vi "Save VI.vi"(8 "error in (no error)":errorcluster, 10 "Ctl Properties":T1[](array[typedef]), 11 "VI Properties":T2) -> (0 "error out":errorcluster, 2 "Saved?":bool, 3 "VI out":refnum<vi>)   [LabVIEW 2023, in "VI Properties Editor.lvlib"]
doc: "Saves a VI based with <B>VI Properties</B> and <B>Ctl Properties</B>."
uses:
  CTLs/VI Properties.ctl
  <vilib>/picture/picture.llb/imagedata.ctl
  CTLs/Control Properties.ctl
  VI Properties Editor.lvlib
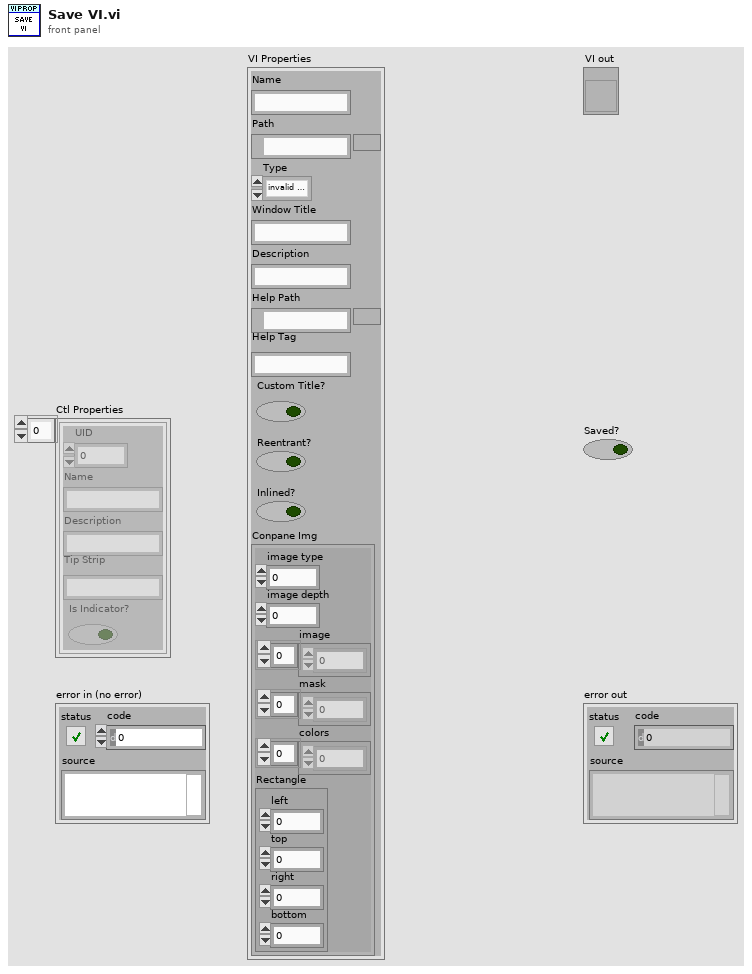
[diagram p1: front panel]
types:
  T1 = typedef "VI Properties Editor.lvlib/Control Properties.ctl" = cluster{"UID":i32, "Name":string, "Description":string, "Tip Strip":string, "Is Indicator?":bool}
  T2 = typedef "VI Properties Editor.lvlib/VI Properties.ctl" = cluster{"Name":string, "Path":path, "Type":enum32{"invalid VI type", "Standard VI", "Control VI", "Global VI", "Polymorphic VI", "Configuration VI", "SubSystem", "Facade VI", "Method VI", "Statechart Diagram VI"}, "Window Title":string, "Description":string, "Help Path":path, "Help Tag":string, "Custom Title?":bool, "Reentrant?":bool, "Inlined?":bool, "Conpane Img":T3}
  T3 = typedef "imagedata.ctl" = cluster{"image type":i32, "image depth":i32, "image":u8[], "mask":u8[], "colors":u32[], "Rectangle":cluster{"left":i16, "top":i16, "right":i16, "bottom":i16}}
  T4 = enum32{"invalid VI type", "Standard VI", "Control VI", "Global VI", "Polymorphic VI", "Configuration VI", "SubSystem", "Facade VI", "Method VI", "Statechart Diagram VI"}
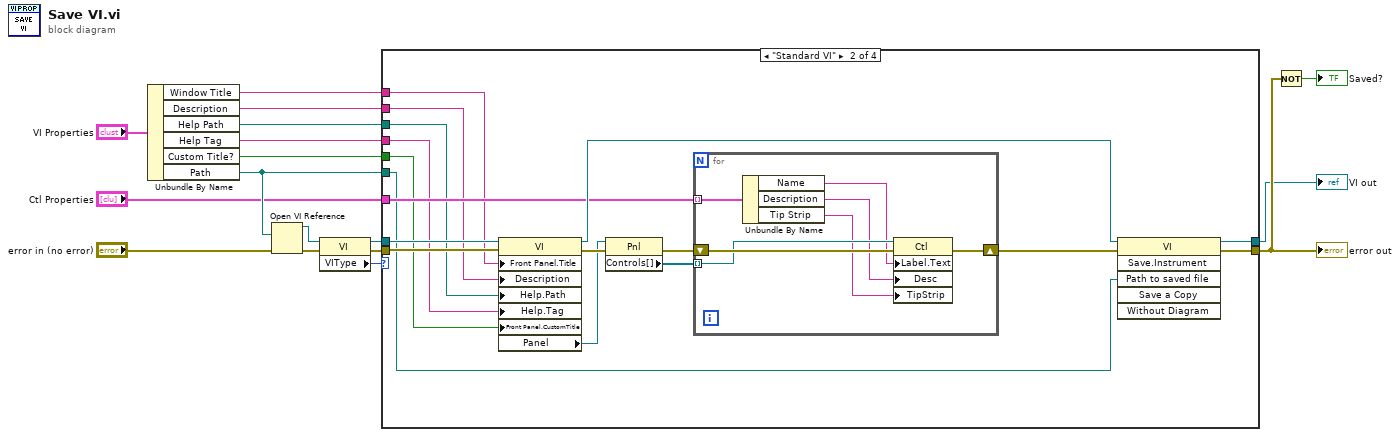
[diagram p0: block diagram]
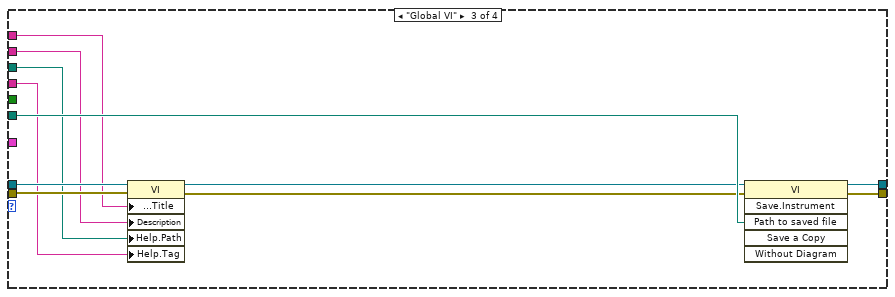
[diagram p3: hidden frame]
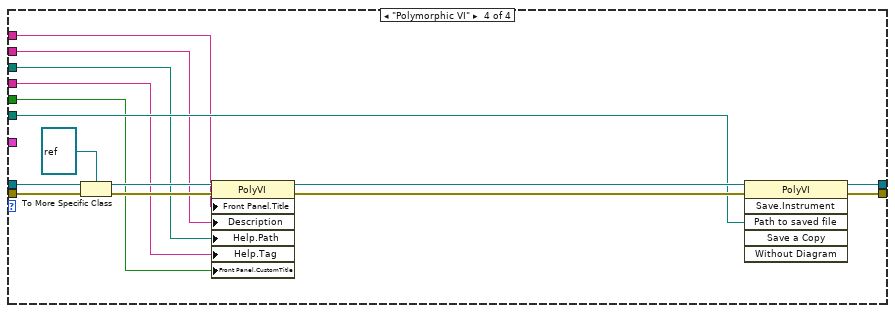
[diagram p4: hidden frame]
diagram:
  n1 = Unbundle By Name("VI Properties") -> ("Window Title"=w2:string, "Description"=w5:string, "Help Path"=w4:path, "Help Tag"=w6:string, "Custom Title?"=w1:bool, "Path"=w7:path)
  n2 = Open VI Reference(vi path=w7, error in (no error)="error in (no error)") -> (vi reference=w10:refnum<vi>, error out=w13:errorcluster)  [unwired: 4 in]
  n3 = property class="VI"(reference=w10, error in=w13) -> (reference out=w11:refnum<vi>, error out=w12:errorcluster, "VIType"=w14:T4)
  n4 = case shown="\"Standard VI\"" w14 {
    tunnel: [w18 w36 w54 w69] -> w15
    tunnel: [w19 w35 w53 w68] -> w16
    tunnel: w11 -> [w18 w28 w49 w66]
    tunnel: w12 -> [w19 w27 w48 w65]
    tunnel: w5 -> [_ w25 w45 w56]
    tunnel: w6 -> [_ w23 w47 w57]
    tunnel: w4 -> [_ w22 w46 w58]
    tunnel: w7 -> [_ w21 w52 w60]
    tunnel: "Ctl Properties" -> [_ w26 _ _]
    tunnel: w2 -> [_ w24 w44 w55]
    tunnel: w1 -> [_ w20 _ w59]
    frame "invalid VI type", Default {
    }
    frame "Standard VI" {
      n5 = property class="VI"(reference=w28, error in=w27, "Front Panel.Title"=w24, "Description"=w25, "Help.Path"=w22, "Help.Tag"=w23, "Front Panel.CustomTitle"=w20) -> (reference out=w31:refnum<vi>, error out=w34:errorcluster, "Panel"=w33:refnum<vi>)
      n6 = property class="Pnl"(reference=w33, error in=w34) -> (error out=w29:errorcluster, "Controls[]"=w30:refnum<vi>[])  [unwired: 1 out]
      n7 = for {
        tunnel: w30 -> [w41] mode=indexing
        shift-right: [w43] -> w32
        shift-left: w29 -> [w42]
        tunnel: w26 -> [w40] mode=indexing
        n8 = Unbundle By Name(w40) -> ("Name"=w39:string, "Description"=w38:string, "Tip Strip"=w37:string)
        n9 = property class="Ctl"(reference=w41, error in=w42, "Label.Text"=w39, "Desc"=w38, "TipStrip"=w37) -> (error out=w43:errorcluster)  [unwired: 1 out]
      }
      n10 = invoke class="VI" method="Save.Instrument"(reference=w31, error in=w32, "Path to saved file"=w21) -> (reference out=w36:refnum<vi>, error out=w35:errorcluster)  [unwired: 3 in, 4 out]
    }
    frame "Global VI" {
      n11 = property class="VI"(reference=w49, error in=w48, "Front Panel.Title"=w44, "Description"=w45, "Help.Path"=w46, "Help.Tag"=w47) -> (reference out=w50:refnum<vi>, error out=w51:errorcluster)
      n12 = invoke class="VI" method="Save.Instrument"(reference=w50, error in=w51, "Path to saved file"=w52) -> (reference out=w54:refnum<vi>, error out=w53:errorcluster)  [unwired: 3 in, 4 out]
    }
    frame "Polymorphic VI" {
      n13 = To More Specific Class(target class=refnum<vi> refnum, reference=w66, error in=w65) -> (specific class reference=w64:refnum<vi>, error out=w63:errorcluster)
      n14 = property class="PolyVI"(reference=w64, error in=w63, "Front Panel.Title"=w55, "Description"=w56, "Help.Path"=w58, "Help.Tag"=w57, "Front Panel.CustomTitle"=w59) -> (reference out=w62:refnum<vi>, error out=w61:errorcluster)
      n15 = invoke class="PolyVI" method="Save.Instrument"(reference=w62, error in=w61, "Path to saved file"=w60) -> (reference out=w69:refnum<vi>, error out=w68:errorcluster)  [unwired: 3 in, 4 out]
    }
  }
  "error out" <- w16
  "VI out" <- w15
  n16 = Not(x=w16) -> (.not. x?=→"Saved?":bool)
